vi "EZT560-Chamber-Control-Tool.vi"() -> ()   [LabVIEW 2015]
panel:
  out "Status":string
  out "PV  (Process Value)":dbl format="%.2f"
  out "SP  (Set Point)":dbl format="%.2f"
  out "Loop %":dbl format="%.2f"
  in  "STOP":bool
  out "SP":dbl(knob) scale=-65.0..90.0
  out "PV":dbl(knob) scale=-65.0..90.0
  in  "Set Alarm Low SP":dbl=-65.0 format="%.1f"
  in  "Set Alarm High SP":dbl=90.0 format="%.1f"
  in  "Set SP":dbl=25.0 format="%.1f"
  in  "Customer Event Control":T1
  in  "Chamber Event Control":T2
  out "Customer Event Status":T1
  out "Chamber Event Status":T3
  out "Alarm High SP":dbl format="%.1f"
  out "Alarm Low SP":dbl format="%.1f"
  in  "Input Monitor Number":i32=1 min=1 max=5
  in  "Loop Number":i32=1 min=1 max=5
  in  "Unit Address":u8=1
  in  "ALARM SILENCE":bool
  out "Status Monitor Alert":bool
  out "Critical Alarm":bool
  in  "Parity":u16(ring)=2 items=["None", "Odd", "Even", "Mark", "Space"]
  in  "Baud Rate":u32=9600
  in  "VISA Session":refnum<visa-resource-name>="COM1"
  in  "UPDATE":bool
  # "CSZ ZP-Series Thermal Chamber Control Tool"
  # "Rev: 1.1.0 (20221206)"
  # "Note: To enable chamber, place check mark on \"Chamber (event 1)\"\nand click [Update] button. To disable, remove check mark."
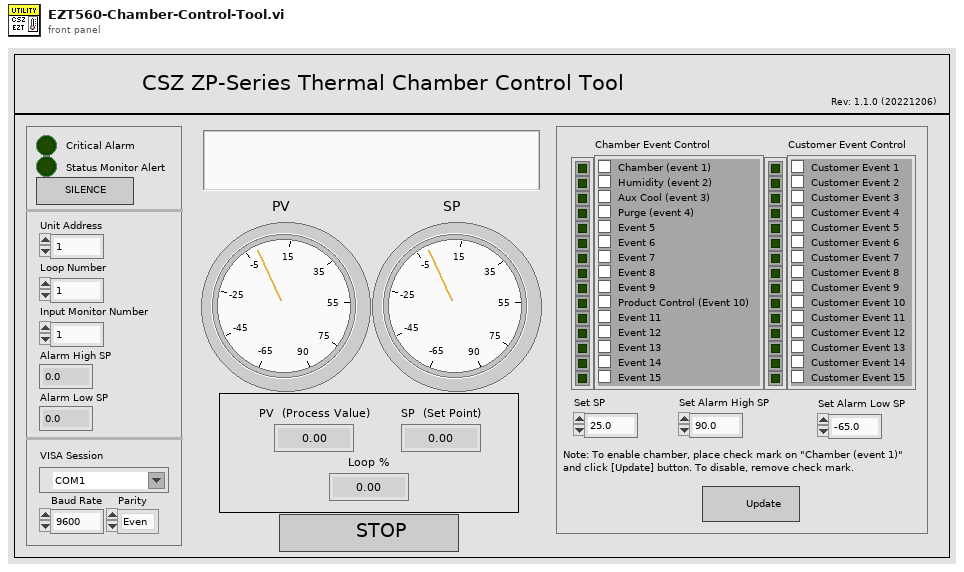
[diagram p1: front panel]
types:
  T1 = cluster{"Customer Event 1":bool, "Customer Event 2":bool, "Customer Event 3":bool, "Customer Event 4":bool, "Customer Event 5":bool, "Customer Event 6":bool, "Customer Event 7":bool, "Customer Event 8":bool, "Customer Event 9":bool, "Customer Event 10":bool, "Customer Event 11":bool, "Customer Event 12":bool, "Customer Event 13":bool, "Customer Event 14":bool, "Customer Event 15":bool}
  T2 = cluster{"Chamber (event 1)":bool, "Humidity (event 2)":bool, "Aux Cool (event 3)":bool, "Purge (event 4)":bool, "Event 5":bool, "Event 6":bool, "Event 7":bool, "Event 8":bool, "Event 9":bool, "Product Control (Event 10)":bool, "Event 11":bool, "Event 12":bool, "Event 13":bool, "Event 14":bool, "Event 15":bool}
  T3 = cluster{"Chamber (event 1)":bool, "Humidity (event 2)":bool, "Aux Cool (event 3)":bool, "Purge (event 4)":bool, "Event 5":bool, "Event 6":bool, "Event 7":bool, "Event 8":bool, "Event 9":bool, "Event 10":bool, "Event 11":bool, "Event 12":bool, "Event 13":bool, "Event 14":bool, "Event 15":bool}
  T4 = enum32{"Invalid", "Standard", "Closed", "Hidden", "Minimized", "Maximized"}
  T5 = enum32{"invalid app kind", "Development System", "Run Time System", "Student Edition", "Embedded LabVIEW", "Evaluation", "Custom"}
  T6 = cluster{"Alarm Type":enum16{"Off", "Process High", "Process Low", "Process Both", "Deviation High", "Deviation Low", "Deviation Both"}, "Alarm Mode Status":cluster{"Alarm Latching":bool, "Output Action":bool, "Audible":bool, "Chamber Action":bool}, "Alarm Output Assigned":enum16{"None", "Customer Event 1", "Customer Event 2", "Customer Event 3", "Customer Event 4", "Customer Event 5", "Customer Event 6", "Customer Event 7", "Customer Event 8", "Customer Event 9", "Customer Event 10", "Customer Event 11", "Customer Event 12", "Customer Event 13", "Customer Event 14", "Customer Event 15"}, "Alarm High Setpoint":dbl, "Alarm Low Setpoint":dbl, "Hysteresis":dbl}
  T7 = cluster{"Core":cluster{"Current VI Reference":refnum<vi>, "Close Panel on Exit?":bool}, "Status":string, "dup VISA session":refnum<visa-resource-name>, "Unit Address":u8, "Loop Number":i32, "Current Alarm Configuration":cluster{"Alarm Type":enum16{"Off", "Process High", "Process Low", "Process Both"}, "Alarm Mode Status":cluster{"Alarm Latching":bool, "Output Action":bool, "Audible":bool, "Chamber Action":bool}, "Alarm Output Assigned":enum16{"None", "Customer Event 1", "Customer Event 2", "Customer Event 3", "Customer Event 4", "Customer Event 5", "Customer Event 6", "Customer Event 7", "Customer Event 8", "Customer Event 9", "Customer Event 10", "Customer Event 11", "Customer Event 12", "Customer Event 13", "Customer Event 14", "Customer Event 15"}, "Alarm High Setpoint":dbl, "Alarm Low Setpoint":dbl, "Hysteresis":dbl}, "Input Monitor Number":i32, "Chamber Event Status":cluster{"Chamber (event 1)":bool, "Humidity (event 2)":bool, "Aux Cool (event 3)":bool, "Purge (event 4)":bool, "Event 5":bool, "Event 6":bool, "Event 7":bool, "Event 8":bool, "Event 9":bool, "Event 10":bool, "Event 11":bool, "Event 12":bool, "Event 13":bool, "Event 14":bool, "Event 15":bool}, "Customer Event Status":cluster{"Customer Event 1":bool, "Customer Event 2":bool, "Customer Event 3":bool, "Customer Event 4":bool, "Customer Event 5":bool, "Customer Event 6":bool, "Customer Event 7":bool, "Customer Event 8":bool, "Customer Event 9":bool, "Customer Event 10":bool, "Customer Event 11":bool, "Customer Event 12":bool, "Customer Event 13":bool, "Customer Event 14":bool, "Customer Event 15":bool}}
  T8 = cluster{"Current VI Reference":refnum<vi>, "Close Panel on Exit?":bool}
  T9 = cluster{"Alarm Type":enum16{"Off", "Process High", "Process Low", "Process Both"}, "Alarm Mode Status":cluster{"Alarm Latching":bool, "Output Action":bool, "Audible":bool, "Chamber Action":bool}, "Alarm Output Assigned":enum16{"None", "Customer Event 1", "Customer Event 2", "Customer Event 3", "Customer Event 4", "Customer Event 5", "Customer Event 6", "Customer Event 7", "Customer Event 8", "Customer Event 9", "Customer Event 10", "Customer Event 11", "Customer Event 12", "Customer Event 13", "Customer Event 14", "Customer Event 15"}, "Alarm High Setpoint":dbl, "Alarm Low Setpoint":dbl, "Hysteresis":dbl}
  T10 = enum16{"Off", "Process High", "Process Low", "Process Both"}
  T11 = cluster{"Alarm Latching":bool, "Output Action":bool, "Audible":bool, "Chamber Action":bool}
  T12 = enum16{"None", "Customer Event 1", "Customer Event 2", "Customer Event 3", "Customer Event 4", "Customer Event 5", "Customer Event 6", "Customer Event 7", "Customer Event 8", "Customer Event 9", "Customer Event 10", "Customer Event 11", "Customer Event 12", "Customer Event 13", "Customer Event 14", "Customer Event 15"}
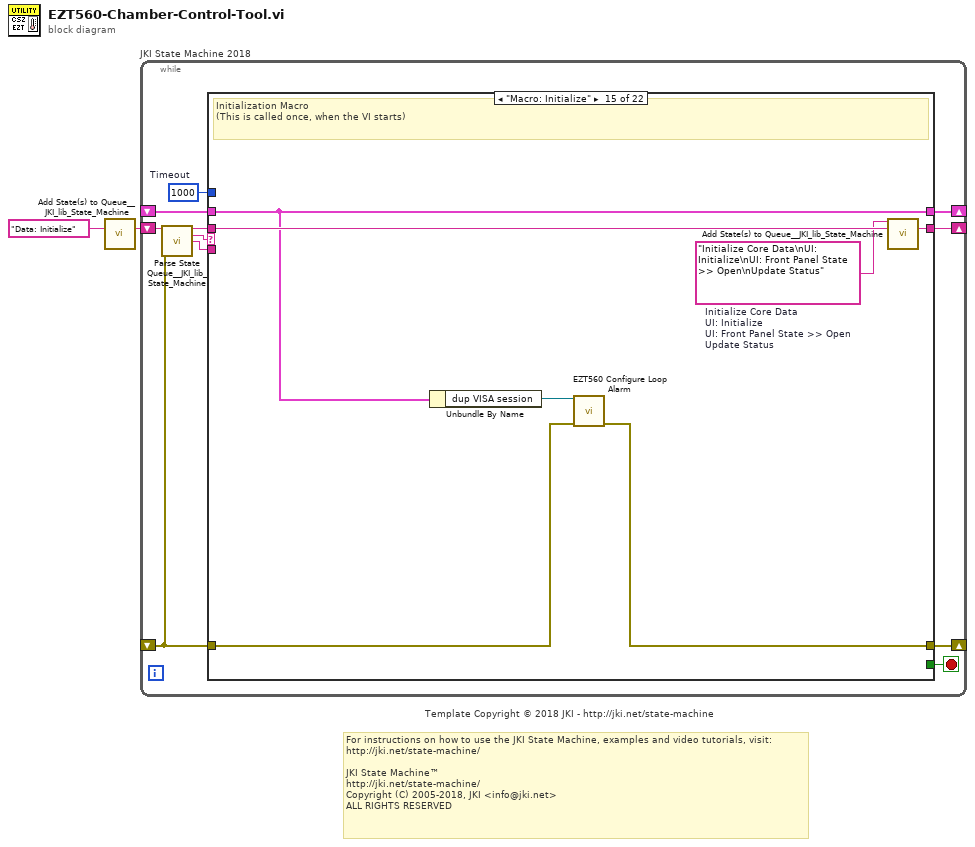
[diagram p0: block diagram]
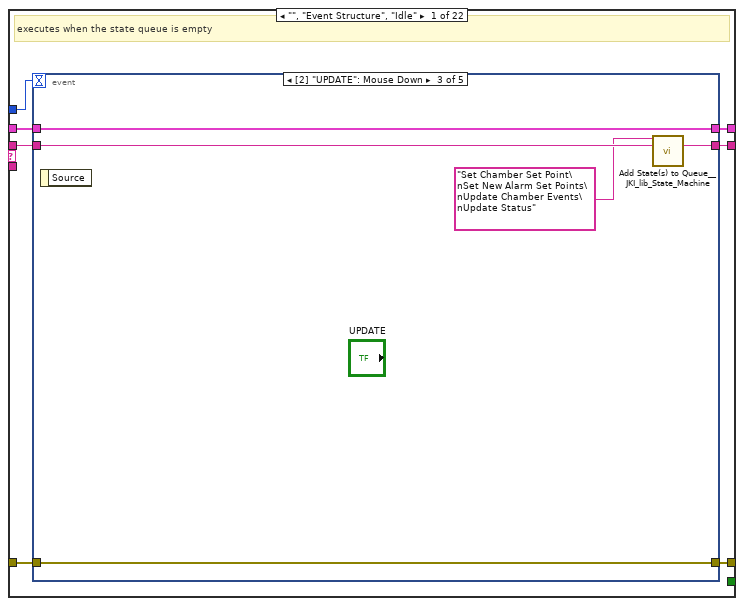
[diagram p2: hidden frame]
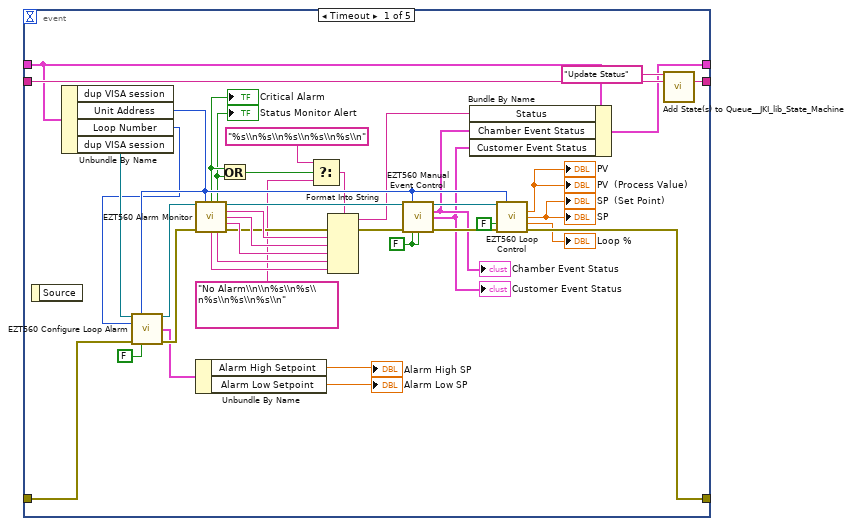
[diagram p3: hidden frame]
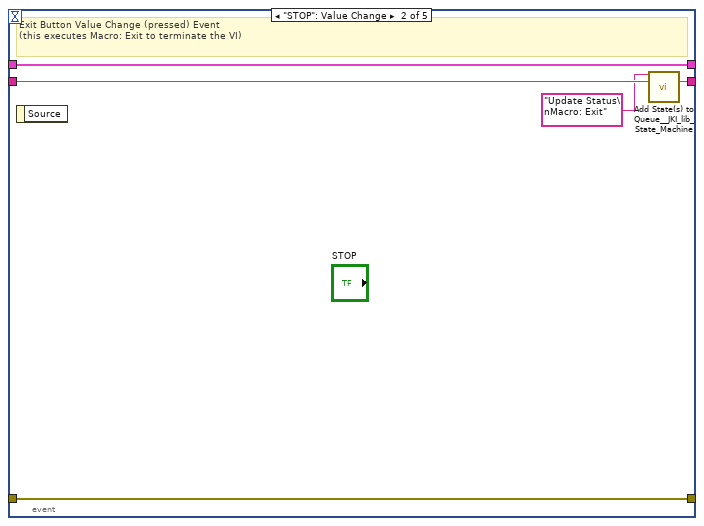
[diagram p4: hidden frame]
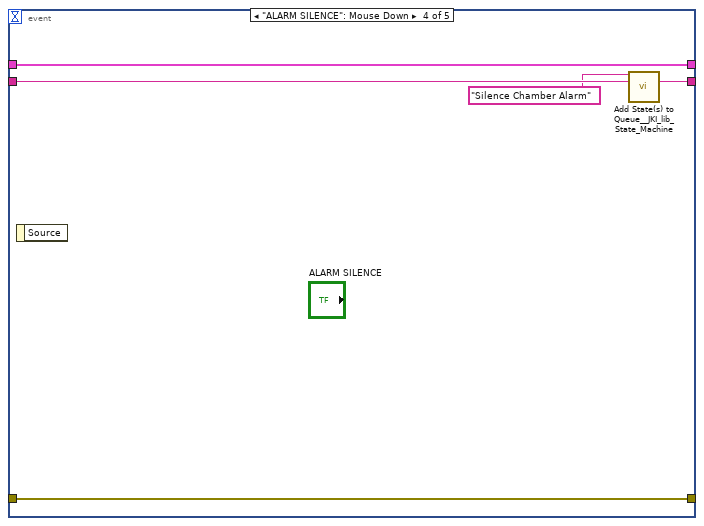
[diagram p5: hidden frame]
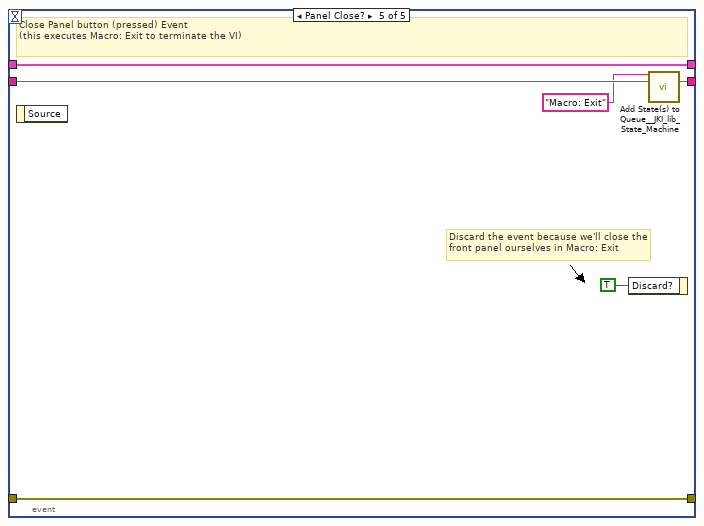
[diagram p6: hidden frame]
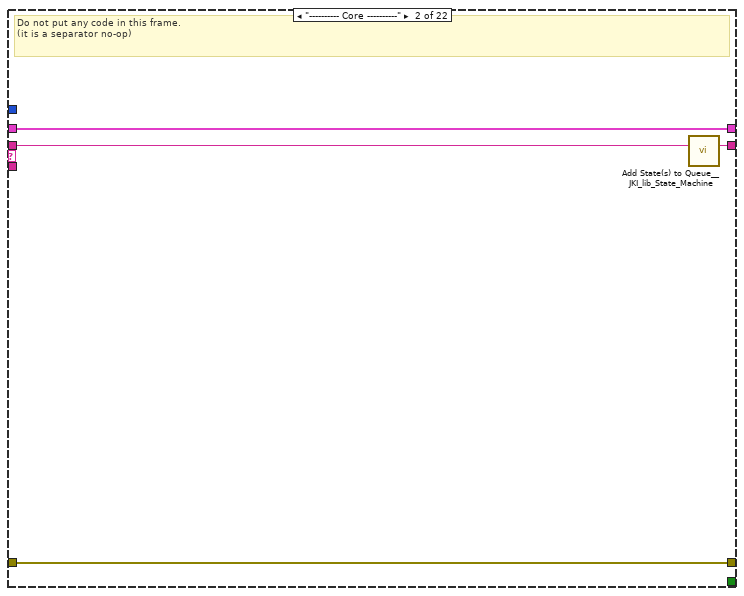
[diagram p7: hidden frame]
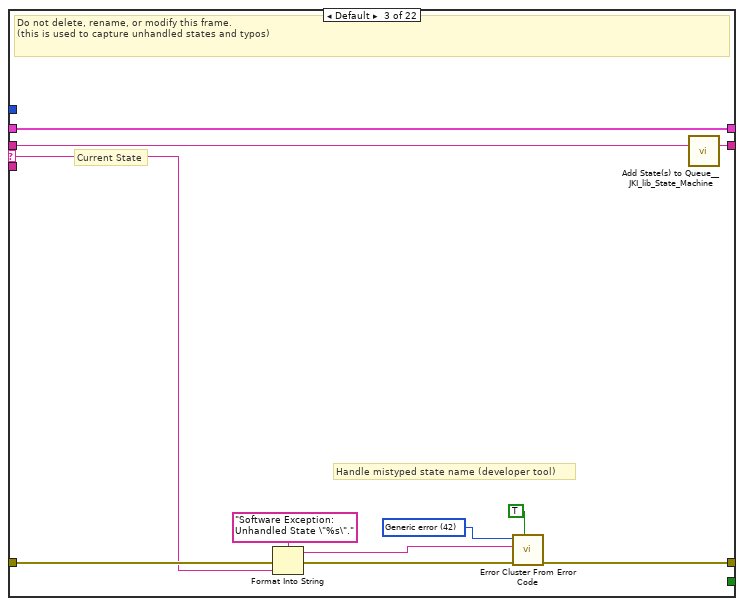
[diagram p8: hidden frame]
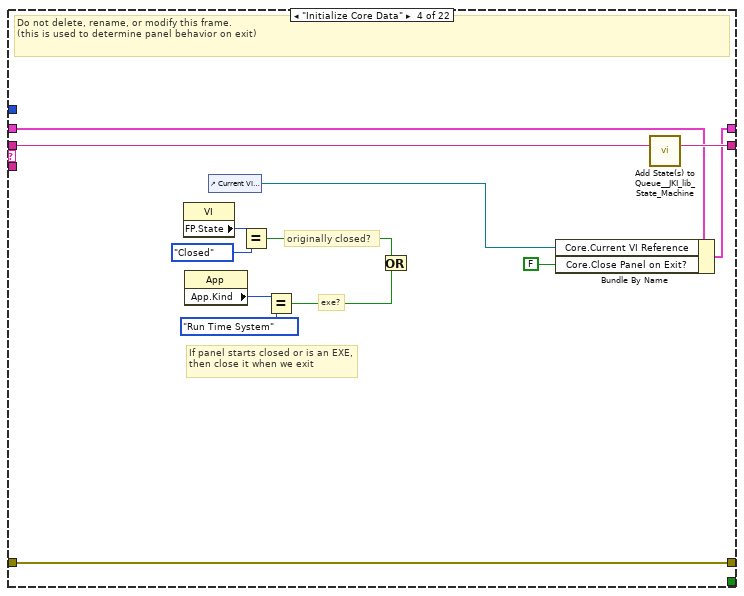
[diagram p9: hidden frame]
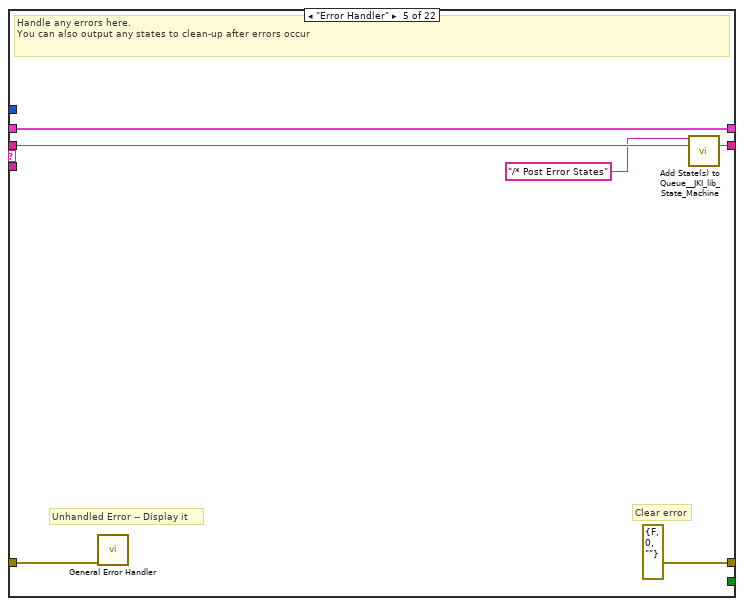
[diagram p10: hidden frame]
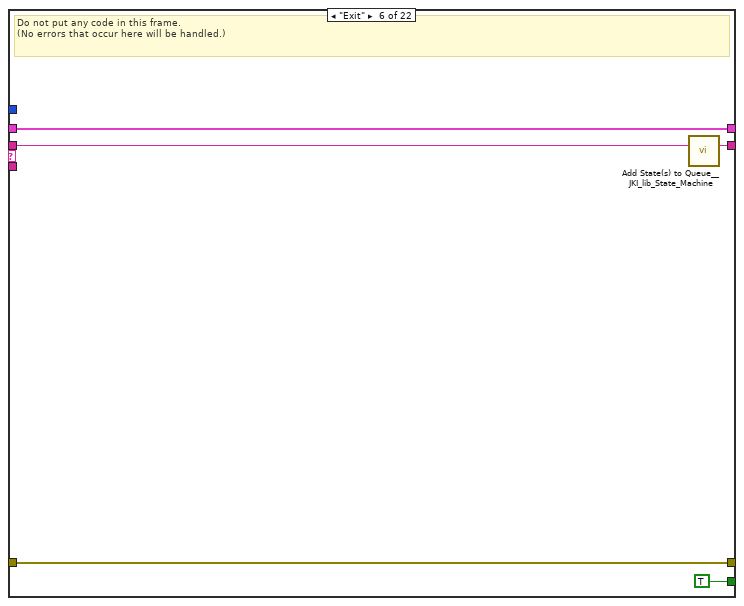
[diagram p11: hidden frame]
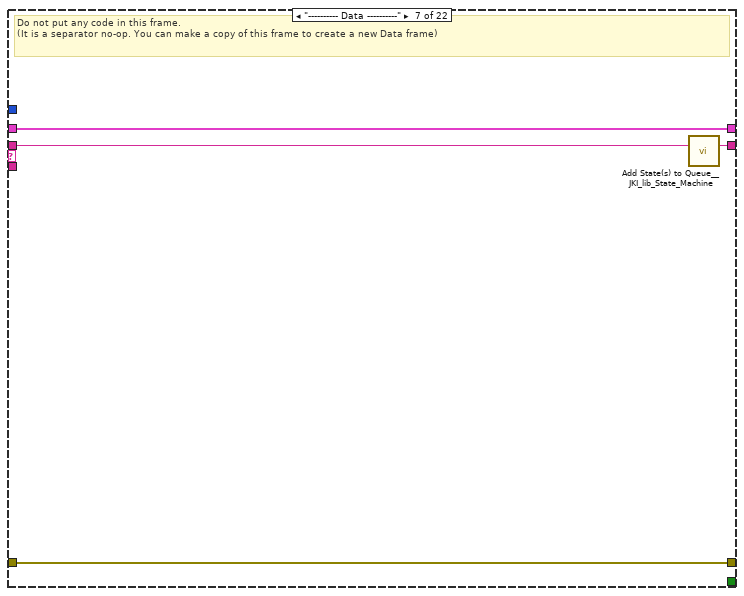
[diagram p12: hidden frame]
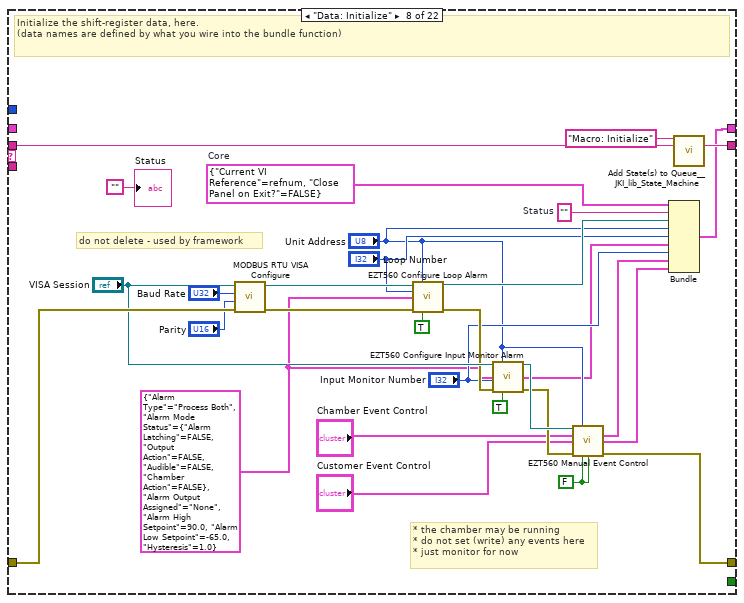
[diagram p13: hidden frame]
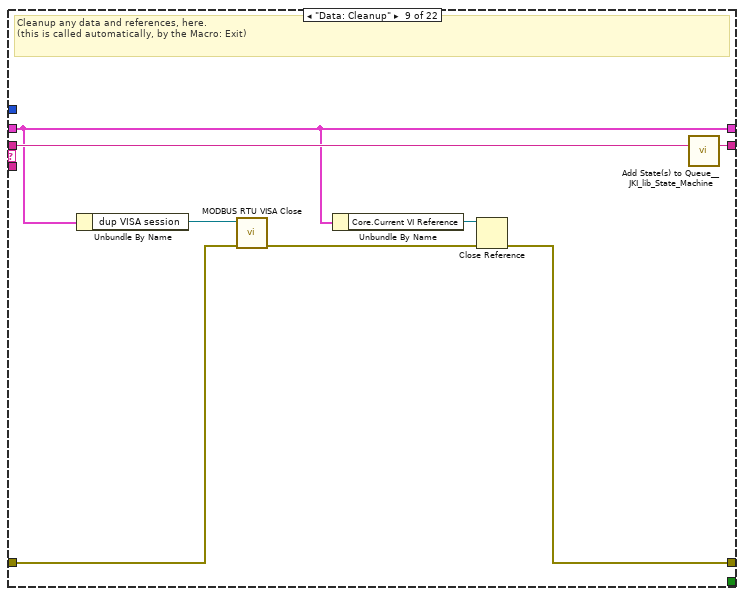
[diagram p14: hidden frame]
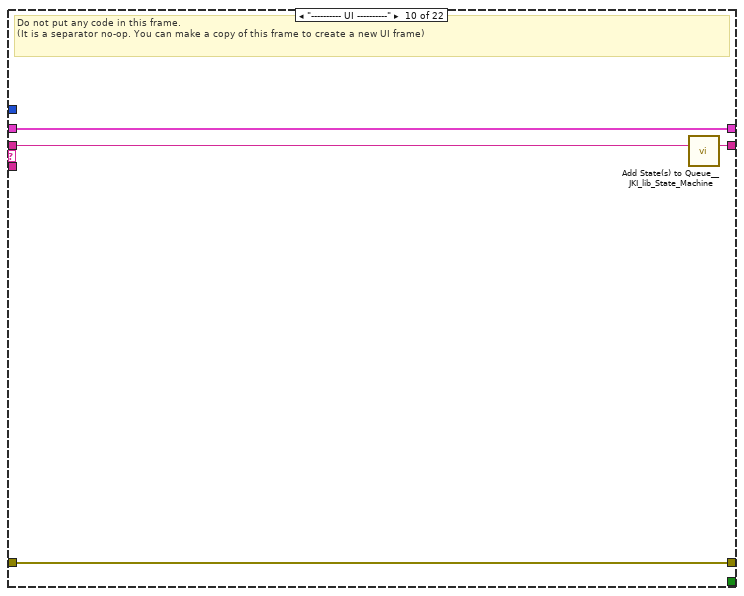
[diagram p15: hidden frame]
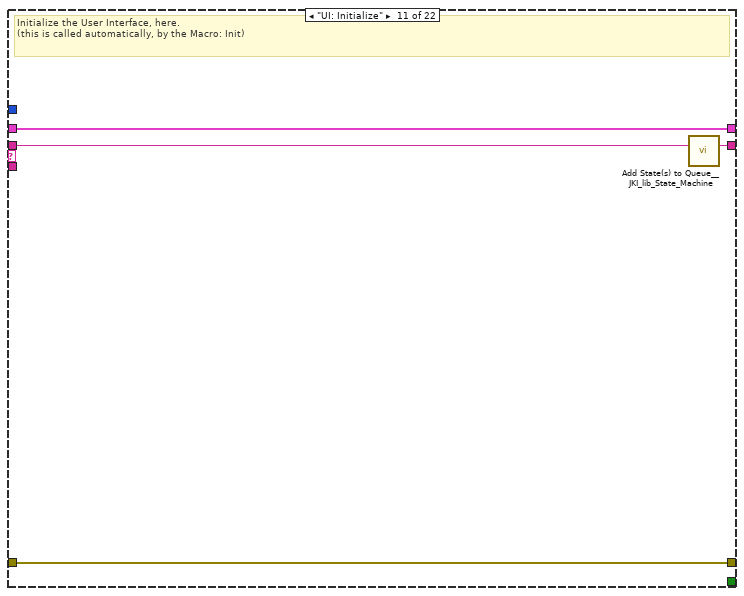
[diagram p16: hidden frame]
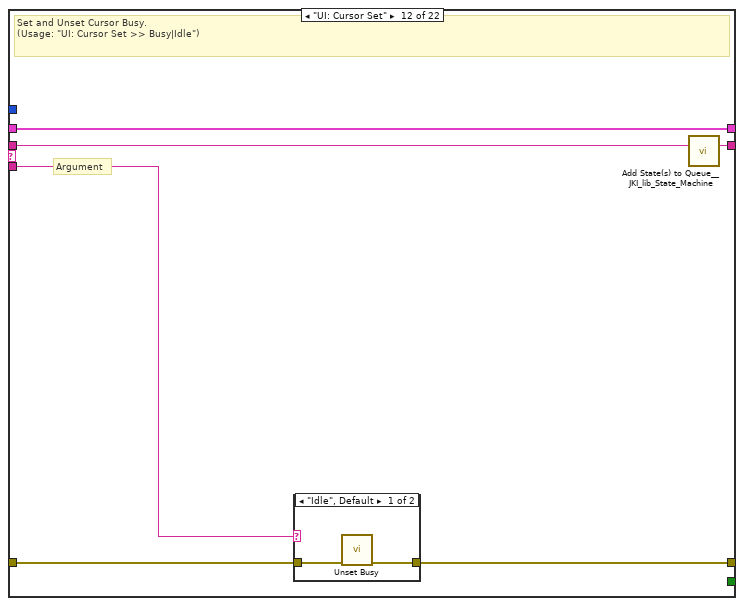
[diagram p17: hidden frame]
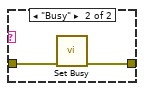
[diagram p18: hidden frame]
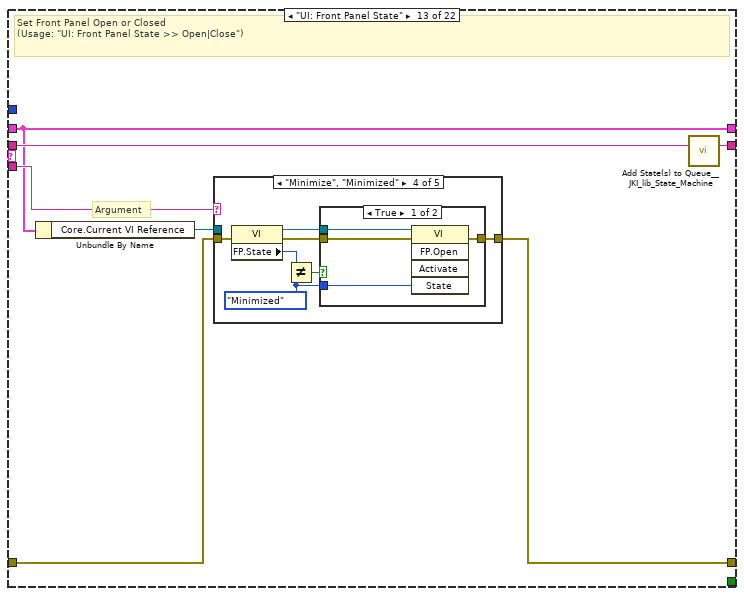
[diagram p19: hidden frame]
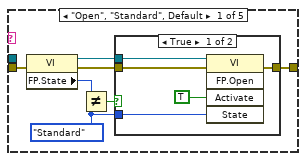
[diagram p20: hidden frame]
diagram:
  # "Template Copyright © 2018 JKI - http://jki.net/state-machine"
  # "For instructions on how to use the JKI State Machine, examples and video tutorials, visit:\nhttp://jki.net/state-machine/\n\nJKI State Machine™\nhttp://jki.net/state-machine/\nCopyright (C) 2005-2018, JKI <info@jki.net>\nALL RIGHTS RESERVED"
  n1 = call <vilib>:"Add State(s) to Queue__JKI_lib_State_Machine.vi"("State(s) in (\"\")"="Data: Initialize") -> ("States Out"=w2:string)  [unwired: 14 in]
  n2 = while "JKI State Machine 2018" {
    shift-right: [w6] -> _
    shift-left: _ -> [w5]
    shift-right: [w9] -> _
    shift-left: _ -> [w3]
    shift-right: [w8] -> _
    shift-left: w2 -> [w10]
    stop <- w7 stop-if-true
    w4 = 1000  # Timeout
    n3 = call <vilib>:"Parse State Queue__JKI_lib_State_Machine.vi"("State Queue"=w10, "Error In (no error)"=w3) -> ("Remaining States"=w12:string, "Current State"=w13:string, "Arguments"=w11:string)  [unwired: 11 in]
    n4 = case shown="\"Macro: Initialize\"" w13 {
      selector: w13 -> [_ _ w86 _ _ _ _ _ _ _ _ _ _ _ _ _ _ _ _ _ _ _]
      tunnel: w12 -> [w20 w85 w90 w109 w115 w120 w124 w154 w162 w166 w170 w176 w187 w251 w258 w268 w272 w283 w310 w323 w345 w358]
      tunnel: w11 -> [_ _ _ _ _ _ _ _ _ _ _ w171 w182 _ _ _ _ _ _ _ _ _]
      tunnel: w5 -> [w18 w82 w88 w99 w112 w118 w121 _ w157 w163 w168 w174 w181 w248 w255 w260 w269 w273 w293 w312 w338 w351]
      tunnel: [w17 w83 w92 w107 errorcluster {"status"=FALSE, "code"=0, "source"=""} ("error out") w117 w122 w134 w160 w164 w167 w172 w184 w249 w253 w266 w270 w281 w296 w320 w342 w354] -> w9
      tunnel: w3 -> [w16 w83 w91 w107 w111 w117 w122 w150 w159 w164 w167 w173 w185 w249 w254 w266 w270 w281 w297 w321 w343 w355]
      tunnel: [w19 w84 w89 w108 w114 w119 w123 w153 w161 w165 w169 w175 w186 w250 w257 w267 w271 w282 w309 w322 w344 w357] -> w8
      tunnel: [_ _ _ _ _ TRUE _ _ _ _ _ _ _ _ _ _ _ _ _ _ _ _] -> w7
      tunnel: [w15 w82 w88 w98 w112 w118 w121 w151 w157 w163 w168 w174 w181 w248 w255 w260 w269 w273 w294 w311 w337 w350] -> w6
      tunnel: w4 -> [w14 _ _ _ _ _ _ _ _ _ _ _ _ _ _ _ _ _ _ _ _ _]
      frame "", "Event Structure", "Idle" {
        # "executes when the state queue is empty"
        n5 = event shown="[2] \"UPDATE\": Mouse Down" {
          selector: _ -> [_ _ _ _ _]
          dyn-events: _ -> [_ _ _ _ _]
          timeout: w14 -> [_ _ _ _ _]
          tunnel: w20 -> [w60 w65 w69 w73 w81]
          tunnel: [w59 w64 w68 w72 w80] -> w19
          tunnel: w18 -> [w39 w61 w70 w75 w78]
          tunnel: [w58 w63 w66 w74 w79] -> w17
          tunnel: w16 -> [w50 w63 w66 w74 w79]
          tunnel: [w38 w61 w70 w75 w78] -> w15
          event Timeout {
            w21 = FALSE ("Update Chamber Events")
            n6 = event-data() -> ()  [unwired: 1 in, 1 out]
            n7 = Unbundle By Name(w39) -> ("Unit Address"=w47:u8, "Loop Number"=w46:i32, "dup VISA session"=w48:refnum<visa-resource-name>)  [unwired: 1 out]
            n8 = call "EZT560 Configure Loop Alarm.vi"("VISA session"=w48, "Unit Address"=w47, "Loop Number"=w46, "error in (no error)"=w50, "Read/Write Alarm Configuration"=FALSE) -> ("dup VISA session"=w44:refnum<visa-resource-name>, "Current Alarm Configuration"=w43:T6, "error out"=w49:errorcluster)  [unwired: 8 in]
            n9 = call "EZT560 Alarm Monitor.vi"("VISA session"=w44, "Unit Address"=w47, "error in (no error)"=w49) -> ("Critical Alarm"=w28:bool, "Status Monitor Alert"=w27:bool, "dup VISA session"=w51:refnum<visa-resource-name>, "Critical Chamber Alarrm"=w37:string, "Critical Refrigeration Alarm"=w36:string, "Non-Critical Alarrm"=w35:string, "EZT Status Alarm"=w33:string, "Input Alarm"=w34:string, "error out"=w32:errorcluster)  [unwired: 4 in]
            "Critical Alarm" <- w28
            "Status Monitor Alert" <- w27
            n10 = Unbundle By Name(w43) -> ("Alarm High Setpoint"=→"Alarm High SP":dbl, "Alarm Low Setpoint"=→"Alarm Low SP":dbl)
            n11 = Or(x=w28, y=w27) -> (x .or. y?=w26:bool)
            n12 = Select(t="%s\\n%s\\n%s\\n%s\\n%s\\n" ("format string"), s=w26, f="No Alarm\\n\\n%s\\n%s\\n%s\\n%s\\n%s\\n" ("format string")) -> (s? t:f=w25:string)
            n13 = Format Into String(format string=w25, error in=w32, w37, w36, w35, w34, w33) -> (resulting string=w30:string, error out=w31:errorcluster)  [unwired: 1 in]
            n14 = call "EZT560 Manual Event Control.vi"("VISA session"=w51, "Unit Address"=w47, "error in (no error)"=w31, "Update Chamber Events"=w21, "Update Customer Events"=w21) -> ("dup VISA session"=w53:refnum<visa-resource-name>, "Chamber Event Status"=w23:T3, "Customer Event Status"=w22:T1, "error out"=w52:errorcluster)  [unwired: 7 in]
            "Chamber Event Status" <- w23
            "Customer Event Status" <- w22
            n15 = Bundle By Name(cluster=w39, "Status"=w30, "Chamber Event Status"=w23, "Customer Event Status"=w22) -> (w38:T7)
            n16 = call "EZT560 Loop Control.vi"("VISA session"=w53, "Unit Address"=w47, "Enter New Setpoint"=FALSE, "error in (no error)"=w52) -> ("Loop PV  (process value)"=→"PV  (Process Value)" →"PV":dbl, "Loop SP  (current setpoint)"=→"SP  (Set Point)" →"SP":dbl, "Loop %  (percent output)"=→"Loop %":dbl, "error out"=w58:errorcluster)  [unwired: 4 in, 4 out]
            n17 = call <vilib>:"Add State(s) to Queue__JKI_lib_State_Machine.vi"("State(s) in Front (\"\")"="Update Status" ("State(s) in Front (\"\")"), "State(s) in (\"\")"=w60) -> ("States Out"=w59:string)  [unwired: 13 in]
          }
          event "STOP": Value Change {
            # "Exit Button Value Change (pressed) Event\n(this executes Macro: Exit to terminate the VI)"
            n18 = event-data() -> ()  [unwired: 1 in, 1 out]
            n19 = call <vilib>:"Add State(s) to Queue__JKI_lib_State_Machine.vi"("State(s) in Front (\"\")"="Update Status\nMacro: Exit", "State(s) in (\"\")"=w65) -> ("States Out"=w64:string)  [unwired: 13 in]
          }
          event "UPDATE": Mouse Down {
            n20 = event-data() -> ()  [unwired: 1 in, 1 out]
            n21 = call <vilib>:"Add State(s) to Queue__JKI_lib_State_Machine.vi"("State(s) in Front (\"\")"="Set Chamber Set Point\nSet New Alarm Set Points\nUpdate Chamber Events\nUpdate Status" ("State(s) in Front (\"\")"), "State(s) in (\"\")"=w69) -> ("States Out"=w68:string)  [unwired: 13 in]
          }
          event "ALARM SILENCE": Mouse Down {
            n22 = event-data() -> ()  [unwired: 1 in, 1 out]
            n23 = call <vilib>:"Add State(s) to Queue__JKI_lib_State_Machine.vi"("State(s) in Front (\"\")"="Silence Chamber Alarm" ("State(s) in Front (\"\")"), "State(s) in (\"\")"=w73) -> ("States Out"=w72:string)  [unwired: 13 in]
          }
          event Panel Close? {
            # "Discard the event because we'll close the front panel ourselves in Macro: Exit"
            # "Close Panel button (pressed) Event\n(this executes Macro: Exit to terminate the VI)"
            n24 = event-data() -> ()  [unwired: 1 in, 1 out]
            n25 = event-data("Discard?"=TRUE) -> ()  [unwired: 1 in, 1 out]
            n26 = call <vilib>:"Add State(s) to Queue__JKI_lib_State_Machine.vi"("State(s) in Front (\"\")"="Macro: Exit", "State(s) in (\"\")"=w81) -> ("States Out"=w80:string)  [unwired: 13 in]
          }
        }
      }
      frame "---------- Core ----------" {
        # "Do not put any code in this frame.\n(it is a separator no-op)"
        n27 = call <vilib>:"Add State(s) to Queue__JKI_lib_State_Machine.vi"("State(s) in (\"\")"=w85) -> ("States Out"=w84:string)  [unwired: 14 in]
      }
      frame Default {
        w95 = 42 items=["No error", "Argument error", "Memory is full", "Out of zone", "End of file", "File already open", "Generic file I/O error", "File not found", "File permission error", "Disk is full", "Duplicate path", "Too many files open", "System feature not enabled", "Resource file not found", "Cannot add resource", "Resource not found", "Image not found", "Image memory error", "Pen does not exist", "Config type invalid", "Config token not found", "Config parse error", "Config memory error", "Bad external code format", "Bad external code offset", "External code not present", "Null window", "Destroy window error", "Null menu", "Print aborted", "Bad print record", "Print driver error", "Windows error during printing", "Memory error during printing", "Print dialog error", "Generic print error", "Invalid device refnum", "Device not found", "Device parameter error", "Device unit error", "Cannot open device", "Device call aborted", "Generic error", "Cancelled by user", "Object ID too low", "Object ID too high", "Object not in heap", "Unknown heap", "Unknown object (invalid DefProc)", "Unknown object (DefProc not in table)", "Message out of range", "Invalid (null) method", "Unknown message", "Manager call not supported", "Bad address", "Network operation in progress", "Network operation timed out", "Connection is busy", "Network attribute not supported", "Network error", "Address in use", "System out of memory", "Connection aborted", "Connection refused", "Not connected", "Already connected", "Connection closed", "Initialization error (interapplication manager)", "Bad occurrence", "Wait on unbound occurrence handler", "Occurrence queue overflow", "Datalog type conflict", "Unused", "Unrecognized type (interapplication manager)", "Memory corrupt", "Failed to make temporary DLL", "Old CIN version", "Drag socket not found", "Failed to load drop-object", "Failed to register OLE object", "Failed to release OLE object", "Format specifier type mismatch", "Unknown format specifier", "Too few format specifiers", "Too many format specifiers", "Scan failed", "Newer CIN version", "Error converting to variant", "Runtime menu error", "Password tampered", "Variant attribute not found", "Incompatible variant data type", "Event data is not available", "Event Store is not present", "Occurrence is not found", "Event Queue is not created", "Event info is not available", "Refnum passed is NULL", "Error retrieving Class GUID", "Error retrieving CoClass GUID", "Error retrieving TypeLib GUID.", "Bad built application magic bytes.", "Specific driver is different from the specific driver associated with the Logical Name.", "There is no session opened to the class driver.", "Max Error", "MAX - Error with config objects", "MAX - Error loading configuration", "MAX - Group not supported"]
        # "Current State"
        # "Handle mistyped state name (developer tool)"
        # "Do not delete, rename, or modify this frame.\n(this is used to capture unhandled states and typos)"
        n28 = Format Into String(format string="Software Exception: Unhandled State \"%s\"." ("message"), error in=w91, w86) -> (resulting string=w94:string, error out=w93:errorcluster)  [unwired: 1 in]
        n29 = call <vilib>:"Error Cluster From Error Code.vi"("show call chain? (False)"=TRUE, "error in (no error)"=w93, "error message (\"\")"=w94, "error code (0)"=w95) -> ("error out"=w92:errorcluster)  [unwired: 5 in]
        n30 = call <vilib>:"Add State(s) to Queue__JKI_lib_State_Machine.vi"("State(s) in (\"\")"=w90) -> ("States Out"=w89:string)  [unwired: 14 in]
      }
      frame "Initialize Core Data" {
        # "originally closed?"
        # "exe?"
        # "If panel starts closed or is an EXE, then close it when we exit"
        # "Do not delete, rename, or modify this frame.\n(this is used to determine panel behavior on exit)"
        n31 = property class="VI"() -> ("FP.State"=w102:T4)  [unwired: 2 in, 2 out]
        n32 = property class="App"() -> ("App.Kind"=w106:T5)  [unwired: 2 in, 2 out]
        n33 = control-ref of="Current VI Reference"() -> (w103:refnum<vi>)
        n34 = Equal?(x=w102, y=T4."Closed" ("Front Panel Window:State")) -> (x = y?=w100:bool)
        n35 = Equal?(x=w106, y=T5."Run Time System" ("Application:Kind")) -> (x = y?=w104:bool)
        n36 = Or(x=w100, y=w104) -> ()  [unwired: 1 out]
        n37 = Bundle By Name(cluster=w99, "Core.Current VI Reference"=w103, "Core.Close Panel on Exit?"=FALSE) -> (w98:T7)
        n38 = call <vilib>:"Add State(s) to Queue__JKI_lib_State_Machine.vi"("State(s) in (\"\")"=w109) -> ("States Out"=w108:string)  [unwired: 14 in]
      }
      frame "Error Handler" {
        # "Unhandled Error -- Display it"
        # "Clear error"
        # "Handle any errors here.\nYou can also output any states to clean-up after errors occur"
        n39 = call <vilib>:"General Error Handler.vi"("error in (no error)"=w111) -> ()  [unwired: 10 in, 5 out]
        n40 = call <vilib>:"Add State(s) to Queue__JKI_lib_State_Machine.vi"("State(s) in Front (\"\")"="/* Post Error States", "State(s) in (\"\")"=w115) -> ("States Out"=w114:string)  [unwired: 13 in]
      }
      frame "Exit" {
        # "Do not put any code in this frame.\n(No errors that occur here will be handled.)"
        n41 = call <vilib>:"Add State(s) to Queue__JKI_lib_State_Machine.vi"("State(s) in (\"\")"=w120) -> ("States Out"=w119:string)  [unwired: 14 in]
      }
      frame "---------- Data ----------" {
        # "Do not put any code in this frame.\n(It is a separator no-op. You can make a copy of this frame to create a new Data frame)"
        n42 = call <vilib>:"Add State(s) to Queue__JKI_lib_State_Machine.vi"("State(s) in (\"\")"=w124) -> ("States Out"=w123:string)  [unwired: 14 in]
      }
      frame "Data: Initialize" {
        w125 = ""  # Status
        w132 = FALSE ("Update Chamber Events")
        w137 = T6 {"Alarm Type"=enum."Process Both", "Alarm Mode Status"={"Alarm Latching"=FALSE, "Output Action"=FALSE, "Audible"=FALSE, "Chamber Action"=FALSE}, "Alarm Output Assigned"=enum."None", "Alarm High Setpoint"=90.0, "Alarm Low Setpoint"=-65.0, "Hysteresis"=1.0} ("New Alarm Configuration")
        w152 = T8 {"Current VI Reference"=refnum, "Close Panel on Exit?"=FALSE}  # Core
        # "* the chamber may be running\n* do not set (write) any events here\n* just monitor for now"
        # "do not delete - used by framework"
        # "Initialize the shift-register data, here.\n(data names are defined by what you wire into the bundle function)"
        n43 = call "MODBUS RTU VISA Configure.vi"("error in (no error)"=w150, "Parity"="Parity", "Baud Rate"="Baud Rate", "VISA Session"="VISA Session") -> ("error out"=w144:errorcluster, "duplicate VISA Session"=w146:refnum<visa-resource-name>)  [unwired: 6 in]
        n44 = call "EZT560 Configure Loop Alarm.vi"("VISA session"=w146, "Unit Address"="Unit Address", "Loop Number"="Loop Number", "New Alarm Configuration"=w137, "error in (no error)"=w144, "Read/Write Alarm Configuration"=TRUE) -> ("dup VISA session"=w145:refnum<visa-resource-name>, "error out"=w140:errorcluster)  [unwired: 7 in, 1 out]
        n45 = call "EZT560 Configure Input Monitor Alarm.vi"("VISA session"="VISA Session", "Unit Address"="Unit Address", "Input Monitor Number"="Input Monitor Number", "New Alarm Configuration"=w137, "error in (no error)"=w140, "Read/Write Alarm Configuration"=TRUE) -> ("dup VISA session"=w136:refnum<visa-resource-name>, "Current Alarm Configuration"=w127:T9, "error out"=w135:errorcluster)  [unwired: 7 in]
        n46 = call "EZT560 Manual Event Control.vi"("VISA session"=w136, "Unit Address"="Unit Address", "Chamber Event Control"="Chamber Event Control", "Customer Event Control"="Customer Event Control", "error in (no error)"=w135, "Update Chamber Events"=w132, "Update Customer Events"=w132) -> ("Chamber Event Status"=w131:T3, "Customer Event Status"=w130:T1, "error out"=w134:errorcluster)  [unwired: 5 in, 1 out]
        n47 = Bundle("Core"=w152, "Status"=w125, "dup VISA session"=w145, "Unit Address"="Unit Address", "Loop Number"="Loop Number", "Current Alarm Configuration"=w127, "Input Monitor Number"="Input Monitor Number", "Chamber Event Status"=w131, "Customer Event Status"=w130) -> (w151:T7)  [unwired: 1 in]
        n48 = call <vilib>:"Add State(s) to Queue__JKI_lib_State_Machine.vi"("State(s) in Front (\"\")"="Macro: Initialize" ("State(s) in Front (\"\")"), "State(s) in (\"\")"=w154) -> ("States Out"=w153:string)  [unwired: 13 in]
        "Status" <- ""
      }
      frame "Data: Cleanup" {
        # "Cleanup any data and references, here.\n(this is called automatically, by the Macro: Exit)"
        n49 = Unbundle By Name(w157) -> ("dup VISA session"=w156:refnum<visa-resource-name>)
        n50 = call "MODBUS RTU VISA Close.vi"("error in (no error)"=w159, "VISA Session"=w156) -> ("error out"=w158:errorcluster)  [unwired: 8 in, 1 out]
        n51 = Unbundle By Name(w157) -> ("Core.Current VI Reference"=w155:refnum<vi>)
        n52 = Close Reference(reference=w155, error in (no error)=w158) -> (error out=w160:errorcluster)
        n53 = call <vilib>:"Add State(s) to Queue__JKI_lib_State_Machine.vi"("State(s) in (\"\")"=w162) -> ("States Out"=w161:string)  [unwired: 14 in]
      }
      frame "---------- UI ----------" {
        # "Do not put any code in this frame.\n(It is a separator no-op. You can make a copy of this frame to create a new UI frame)"
        n54 = call <vilib>:"Add State(s) to Queue__JKI_lib_State_Machine.vi"("State(s) in (\"\")"=w166) -> ("States Out"=w165:string)  [unwired: 14 in]
      }
      frame "UI: Initialize" {
        # "Initialize the User Interface, here.\n(this is called automatically, by the Macro: Init)"
        n55 = call <vilib>:"Add State(s) to Queue__JKI_lib_State_Machine.vi"("State(s) in (\"\")"=w170) -> ("States Out"=w169:string)  [unwired: 14 in]
      }
      frame "UI: Cursor Set" {
        # "Argument"
        # "Set and Unset Cursor Busy.\n(Usage: \"UI: Cursor Set >> Busy|Idle\")"
        n56 = case shown="\"Idle\", Default" w171 {
          tunnel: w173 -> [w178 w180]
          tunnel: [w177 w179] -> w172
          frame "Idle", Default {
            n57 = call <vilib>:"Unset Busy.vi"("error in (no error)"=w178) -> ("error out"=w177:errorcluster)  [unwired: 10 in]
          }
          frame "Busy" {
            n58 = call <vilib>:"Set Busy.vi"("error in (no error)"=w180) -> ("error out"=w179:errorcluster)  [unwired: 9 in, 1 out]
          }
        }
        n59 = call <vilib>:"Add State(s) to Queue__JKI_lib_State_Machine.vi"("State(s) in (\"\")"=w176) -> ("States Out"=w175:string)  [unwired: 14 in]
      }
      frame "UI: Front Panel State" {
        # "Argument"
        # "Set Front Panel Open or Closed\n(Usage: \"UI: Front Panel State >> Open|Close\")"
        n60 = Unbundle By Name(w181) -> ("Core.Current VI Reference"=w183:refnum<vi>)
        n61 = case shown="\"Minimize\", \"Minimized\"" w182 {
          tunnel: w185 -> [w193 w206 w217 w229 w241]
          tunnel: [w194 w207 w218 w230 w242] -> w184
          tunnel: w183 -> [_ _ _ _ _]
          frame "Open", "Standard", Default {
            w188 = T4."Standard" ("State")
            n62 = property class="VI"(error in=w193) -> (reference out=w191:refnum<vi>, error out=w192:errorcluster, "FP.State"=w190:T4)  [unwired: 1 in]
            n63 = Not Equal?(x=w190, y=w188) -> (x != y?=w189:bool)
            n64 = case shown="True" w189 {
              tunnel: [w198 w200] -> w194
              tunnel: w192 -> [w197 w200]
              tunnel: w191 -> [w196 _]
              tunnel: w188 -> [w195 _]
              frame True {
                n65 = invoke class="VI" method="FP.Open"(reference=w196, error in=w197, "Activate"=TRUE, "State"=w195) -> (error out=w198:errorcluster)  [unwired: 1 in, 4 out]
              }
              frame False {
              }
            }
          }
          frame "Close", "Closed" {
            n66 = property class="VI"(error in=w206) -> (reference out=w204:refnum<vi>, error out=w205:errorcluster, "FP.State"=w202:T4)  [unwired: 1 in]
            n67 = Not Equal?(x=w202, y=T4."Closed" ("Front Panel Window:State")) -> (x != y?=w201:bool)
            n68 = case shown="True" w201 {
              tunnel: [w208 w211] -> w207
              tunnel: w205 -> [w208 w210]
              tunnel: w204 -> [_ w209]
              frame False {
              }
              frame True {
                n69 = invoke class="VI" method="FP.Close"(reference=w209, error in=w210) -> (error out=w211:errorcluster)  [unwired: 1 in, 2 out]
              }
            }
          }
          frame "Hidden", "Hide" {
            w212 = T4."Hidden" ("State")
            n70 = property class="VI"(error in=w217) -> (reference out=w215:refnum<vi>, error out=w216:errorcluster, "FP.State"=w214:T4)  [unwired: 1 in]
            n71 = Not Equal?(x=w214, y=w212) -> (x != y?=w213:bool)
            n72 = case shown="True" w213 {
              tunnel: [w222 w223] -> w218
              tunnel: w216 -> [w221 w223]
              tunnel: w215 -> [w220 _]
              tunnel: w212 -> [w219 _]
              frame True {
                n73 = invoke class="VI" method="FP.Open"(reference=w220, error in=w221, "State"=w219) -> (error out=w222:errorcluster)  [unwired: 2 in, 4 out]
              }
              frame False {
              }
            }
          }
          frame "Minimize", "Minimized" {
            w224 = T4."Minimized" ("State")
            n74 = property class="VI"(error in=w229) -> (reference out=w227:refnum<vi>, error out=w228:errorcluster, "FP.State"=w226:T4)  [unwired: 1 in]
            n75 = Not Equal?(x=w226, y=w224) -> (x != y?=w225:bool)
            n76 = case shown="True" w225 {
              tunnel: [w234 w235] -> w230
              tunnel: w228 -> [w233 w235]
              tunnel: w227 -> [w232 _]
              tunnel: w224 -> [w231 _]
              frame True {
                n77 = invoke class="VI" method="FP.Open"(reference=w232, error in=w233, "State"=w231) -> (error out=w234:errorcluster)  [unwired: 2 in, 4 out]
              }
              frame False {
              }
            }
          }
          frame "Maximize", "Maximized" {
            w236 = T4."Maximized" ("State")
            n78 = property class="VI"(error in=w241) -> (reference out=w239:refnum<vi>, error out=w240:errorcluster, "FP.State"=w238:T4)  [unwired: 1 in]
            n79 = Not Equal?(x=w238, y=w236) -> (x != y?=w237:bool)
            n80 = case shown="True" w237 {
              tunnel: [w246 w247] -> w242
              tunnel: w240 -> [w245 w247]
              tunnel: w239 -> [w244 _]
              tunnel: w236 -> [w243 _]
              frame True {
                n81 = invoke class="VI" method="FP.Open"(reference=w244, error in=w245, "State"=w243) -> (error out=w246:errorcluster)  [unwired: 2 in, 4 out]
              }
              frame False {
              }
            }
          }
        }
        n82 = call <vilib>:"Add State(s) to Queue__JKI_lib_State_Machine.vi"("State(s) in (\"\")"=w187) -> ("States Out"=w186:string)  [unwired: 14 in]
      }
      frame "---------- Macro ----------" {
        # "Do not put any code in this frame.\n(It is a separator no-op. You can make a copy of this frame to create a new Macro frame)"
        n83 = call <vilib>:"Add State(s) to Queue__JKI_lib_State_Machine.vi"("State(s) in (\"\")"=w251) -> ("States Out"=w250:string)  [unwired: 14 in]
      }
      frame "Macro: Initialize" {
        w256 = "Initialize Core Data\nUI: Initialize\nUI: Front Panel State >> Open\nUpdate Status"  # Initialize Core Data UI: Initialize UI: Front Panel State >> Open Update Status
        # "Initialization Macro\n(This is called once, when the VI starts)"
        n84 = Unbundle By Name(w255) -> ("dup VISA session"=w252:refnum<visa-resource-name>)
        n85 = call "EZT560 Configure Loop Alarm.vi"("VISA session"=w252, "error in (no error)"=w254) -> ("error out"=w253:errorcluster)  [unwired: 11 in, 2 out]
        n86 = call <vilib>:"Add State(s) to Queue__JKI_lib_State_Machine.vi"("State(s) in Front (\"\")"=w256, "State(s) in (\"\")"=w258) -> ("States Out"=w257:string)  [unwired: 13 in]
      }
      frame "Macro: Exit" {
        # "Exit Macro\n(This is called once, when the VI exits)"
        n87 = Unbundle By Name(w260) -> ("Core.Close Panel on Exit?"=w259:bool)
        n88 = Select(t="UI: Front Panel State >> Close", s=w259, f="") -> (s? t:f=w263:string)
        n89 = call <vilib>:"Add State(s) to Queue__JKI_lib_State_Machine.vi"("State(s) in (\"\")"=w263, "State(s) at Back (\"\")"="Data: Cleanup\nExit") -> ("States Out"=w261:string)  [unwired: 13 in]
        n90 = call <vilib>:"Add State(s) to Queue__JKI_lib_State_Machine.vi"("State(s) in Front (\"\")"=w261, "State(s) in (\"\")"=w268) -> ("States Out"=w267:string)  [unwired: 13 in]
      }
      frame "---------- New Category ----------" {
        # "Template Separator\n(You can make a copy of, or modify, this frame)"
        n91 = call <vilib>:"Add State(s) to Queue__JKI_lib_State_Machine.vi"("State(s) in (\"\")"=w272) -> ("States Out"=w271:string)  [unwired: 14 in]
      }
      frame "Update Status" {
        # "Template Separator\n(You can make a copy of, or modify, this frame)"
        n92 = Unbundle By Name(w273) -> ("Chamber Event Status.Chamber (event 1)"=w278:bool)
        n93 = Unbundle By Name(w273) -> ("Status"=w275:string)
        n94 = Select(t="CSZ Status: Chamber ON" ("Status"), s=w278, f="CSZ Status: Chamber OFF" ("Status")) -> (s? t:f=w276:string)
        n95 = Concatenate Strings(w276, "\r", w275) -> (w277:string)
        n96 = local write "Status"(w277) -> ()
        n97 = call <vilib>:"Add State(s) to Queue__JKI_lib_State_Machine.vi"("State(s) in (\"\")"=w283) -> ("States Out"=w282:string)  [unwired: 14 in]
      }
      frame "Set New Alarm Set Points" {
        # "Update Loop Alarm Configuration"
        n98 = Unbundle By Name(w293) -> ("Unit Address"=w307:u8, "dup VISA session"=w308:refnum<visa-resource-name>, "Loop Number"=w298:i32, "Current Alarm Configuration"=w306:T9)
        n99 = Unbundle(w306) -> ("Alarm Type"=w300:T10, "Alarm Mode Status"=w301:T11, "Alarm Output Assigned"=w302:T12, "Hysteresis"=w303:dbl)  [unwired: 2 out]
        n100 = Bundle(cluster=w306, "Alarm Type"=w300, "Alarm Mode Status"=w301, "Alarm Output Assigned"=w302, "Alarm High Setpoint"="Set Alarm High SP", "Alarm Low Setpoint"="Set Alarm Low SP", "Hysteresis"=w303) -> (w299:T9)
        n101 = call "EZT560 Configure Loop Alarm.vi"("VISA session"=w308, "Unit Address"=w307, "Loop Number"=w298, "New Alarm Configuration"=w299, "error in (no error)"=w297, "Read/Write Alarm Configuration"=TRUE) -> ("Current Alarm Configuration"=w287:T6, "error out"=w296:errorcluster)  [unwired: 7 in, 1 out]
        n102 = Unbundle(w293) -> ("Core"=w292:T8, "dup VISA session"=w291:refnum<visa-resource-name>, "Unit Address"=w290:u8, "Loop Number"=w286:i32, "Input Monitor Number"=w289:i32, "Chamber Event Status"=w288:T3)  [unwired: 3 out]
        n103 = Bundle(cluster=w293, "Core"=w292, "Status"="CSZ Status: New Alarm High & Low Set" ("format string"), "dup VISA session"=w291, "Unit Address"=w290, "Loop Number"=w286, "Current Alarm Configuration"=w287, "Input Monitor Number"=w289, "Chamber Event Status"=w288) -> (w294:T7)  [unwired: 1 in]
        n104 = call <vilib>:"Add State(s) to Queue__JKI_lib_State_Machine.vi"("State(s) in Front (\"\")"="Update Status" ("State(s) in Front (\"\")"), "State(s) in (\"\")"=w310) -> ("States Out"=w309:string)  [unwired: 13 in]
      }
      frame "Set Chamber Set Point" {
        w315 = TRUE ("Enter New Setpoint")
        n105 = Unbundle By Name(w312) -> ("Unit Address"=w318:u8, "dup VISA session"=w319:refnum<visa-resource-name>, "Loop Number"=w317:i32)
        n106 = call "EZT560 Loop Control.vi"("VISA session"=w319, "Unit Address"=w318, "Loop Number"=w317, "New Loop Setpoint"="Set SP", "Enter New Setpoint"=w315, "error in (no error)"=w321, "Initiate Tune"=w315) -> ("error out"=w320:errorcluster)  [unwired: 1 in, 7 out]
        n107 = Bundle By Name(cluster=w312, "Status"="CSZ Status: New Set Points Enabled" ("format string")) -> (w311:T7)
        n108 = call <vilib>:"Add State(s) to Queue__JKI_lib_State_Machine.vi"("State(s) in Front (\"\")"="Update Status" ("State(s) in Front (\"\")"), "State(s) in (\"\")"=w323) -> ("States Out"=w322:string)  [unwired: 13 in]
      }
      frame "Silence Chamber Alarm" {
        w339 = TRUE ("Alarm Acknowledge")
        # "Template Separator\n(You can make a copy of, or modify, this frame)"
        n109 = Unbundle By Name(w338) -> ("Unit Address"=w340:u8, "dup VISA session"=w341:refnum<visa-resource-name>)
        n110 = call "EZT560 Alarm Monitor.vi"("VISA session"=w341, "Unit Address"=w340, "Alarm Acknowledge"=w339, "Pumpdown Enable"=w339, "error in (no error)"=w343) -> ("Critical Alarm"=w328:bool, "Status Monitor Alert"=w329:bool, "Critical Chamber Alarrm"=w336:string, "Critical Refrigeration Alarm"=w335:string, "Non-Critical Alarrm"=w334:string, "EZT Status Alarm"=w332:string, "Input Alarm"=w333:string, "error out"=w342:errorcluster)  [unwired: 2 in, 1 out]
        n111 = Or(x=w328, y=w329) -> (x .or. y?=w327:bool)
        n112 = Select(t="CSZ Status:\\n%s\\n%s\\n%s\\n%s\\n%s\\n" ("format string"), s=w327, f="CSZ Status: No Alarm\\n\\n%s\\n%s\\n%s\\n%s\\n%s\\n" ("format string")) -> (s? t:f=w325:string)
        n113 = Format Into String(format string=w325, w336, w335, w334, w333, w332) -> (resulting string=w331:string)  [unwired: 2 in, 1 out]
        n114 = Bundle By Name(cluster=w338, "Status"=w331) -> (w337:T7)
        n115 = call <vilib>:"Add State(s) to Queue__JKI_lib_State_Machine.vi"("State(s) in Front (\"\")"="Update Status" ("State(s) in Front (\"\")"), "State(s) in (\"\")"=w345) -> ("States Out"=w344:string)  [unwired: 13 in]
      }
      frame "Update Chamber Events" {
        w347 = TRUE ("Update Chamber Events")
        # "Update Chamber/Customer Events"
        n116 = local read "Customer Event Control"() -> (w352:T1)
        n117 = Unbundle By Name(w351) -> ("Unit Address"=w346:u8, "dup VISA session"=w356:refnum<visa-resource-name>)
        n118 = local read "Chamber Event Control"() -> (w353:T2)
        n119 = call "EZT560 Manual Event Control.vi"("VISA session"=w356, "Unit Address"=w346, "Chamber Event Control"=w353, "Customer Event Control"=w352, "error in (no error)"=w355, "Update Chamber Events"=w347, "Update Customer Events"=w347) -> ("Chamber Event Status"=w349:T3, "Customer Event Status"=w348:T1, "error out"=w354:errorcluster)  [unwired: 5 in, 1 out]
        n120 = Bundle By Name(cluster=w351, "Chamber Event Status"=w349, "Customer Event Status"=w348) -> (w350:T7)
        n121 = call <vilib>:"Add State(s) to Queue__JKI_lib_State_Machine.vi"("State(s) in (\"\")"=w358) -> ("States Out"=w357:string)  [unwired: 14 in]
      }
    }
  }
